vi "Initialize.vi"(8 "error in (no error)":errorcluster, 11 "Master in":refnum<class "Master.lvclass">) -> (0 "error out":errorcluster, 3 "Master out":refnum<class "Master.lvclass">)   [LabVIEW 2014, in "Master.lvclass"]
uses:
  Master.lvclass
  Controls/StateDatas.ctl
  Master.lvclass/Master.ctl
  Controls/Control Library.lvlib
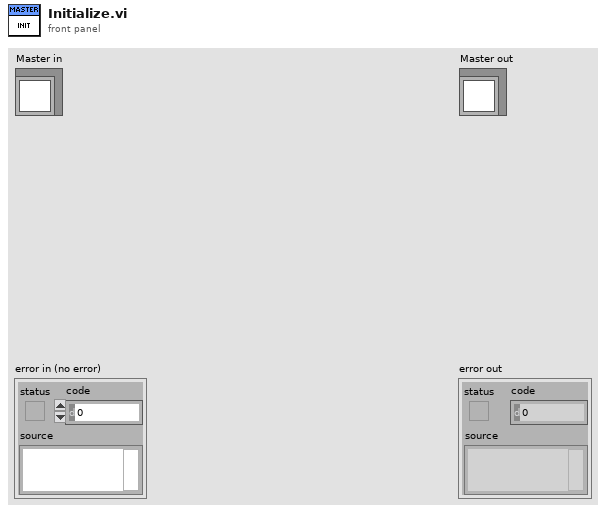
[diagram p1: front panel]
types:
  T1 = typedef "Control Library.lvlib/StateDatas.ctl" = cluster{"State":string, "Data":variant}
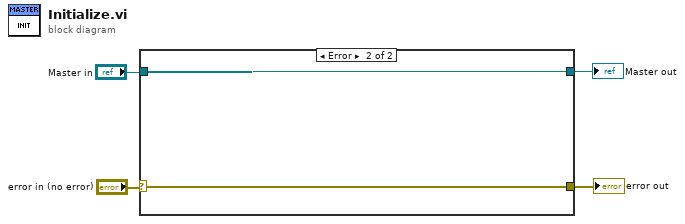
[diagram p0: block diagram]
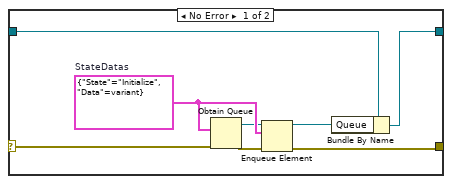
[diagram p2: hidden frame]
diagram:
  n1 = case shown="Error" "error in (no error)" {
    selector: "error in (no error)" -> [w6 w14]
    tunnel: [w9 w14] -> w3
    tunnel: [w8 w13] -> w1
    tunnel: "Master in" -> [w5 w13]
    frame No Error {
      w12 = T1 {"State"="Initialize", "Data"=variant}  # StateDatas
      n2 = Obtain Queue(element data type=w12, error in (no error)=w6) -> (queue out=w10:refnum<queue>, error out=w11:errorcluster)  [unwired: 3 in, 1 out]
      n3 = Enqueue Element(queue=w10, element=w12, error in (no error)=w11) -> (queue out=w7:refnum<queue>, error out=w9:errorcluster)  [unwired: 1 in, 1 out]
      n4 = Bundle By Name(cluster=w5, "Queue"=w7) -> (w8:refnum<class "Master.lvclass">)
    }
    frame Error {
    }
  }
  "error out" <- w3
  "Master out" <- w1
